vi "nonlinearmixpart.vi"(0 "Number of Samples":dbl, 1 "LO Frequency":dbl, 4 "Integer Degree of Nonlinearity (LO) (N) ( y(t) = x^1(t) + ...  + x^N(t) )":i32, 5 "Low Side / High Side":bool, 6 "Sampling Info":cluster{"Numeric 2":dbl, "Numeric":dbl}, 7 "RF Passband Bandwidth (Hz)":dbl, 9 "LO Gain Terms  (first gain term applied to linear part)":dbl[](array[numeric]), 10 "RF Carrier Frequency":dbl, 11 "Show Image Band":bool, 12 "Integer Degree of Nonlinearity (RF) (N) ( y(t) = x^1(t) + ...  + x^N(t) )":i32, 13 "RF Gain Terms (first gain term applied to linear part)":dbl[](array[numeric]), 19 "Duration (Seconds)":dbl) -> (14 "Post Distortion Passband Waveform":waveform(dbl), 15 "Post-distortion Local Oscillator Waveform":waveform(dbl), 17 "Pre-distortion passband waveform":waveform(dbl), 18 "Pre-distortion Local Oscillator Waveform":waveform(dbl))   [LabVIEW 2009]
uses:
  <vilib>/measure/NI_MABase.lvlib
  <vilib>/Analysis/NI_AALBase.lvlib
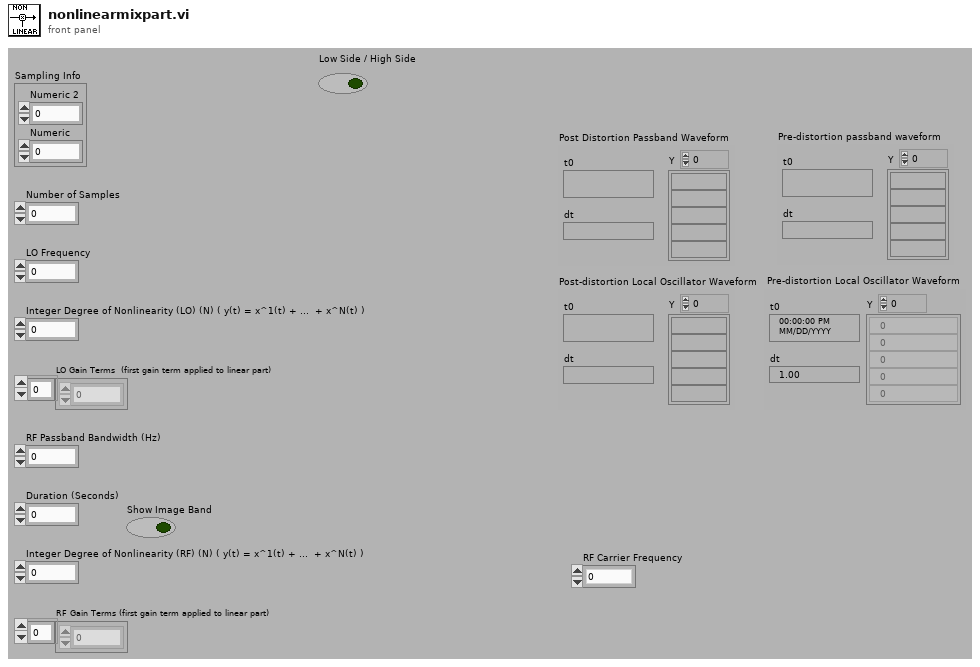
[diagram p1: front panel]
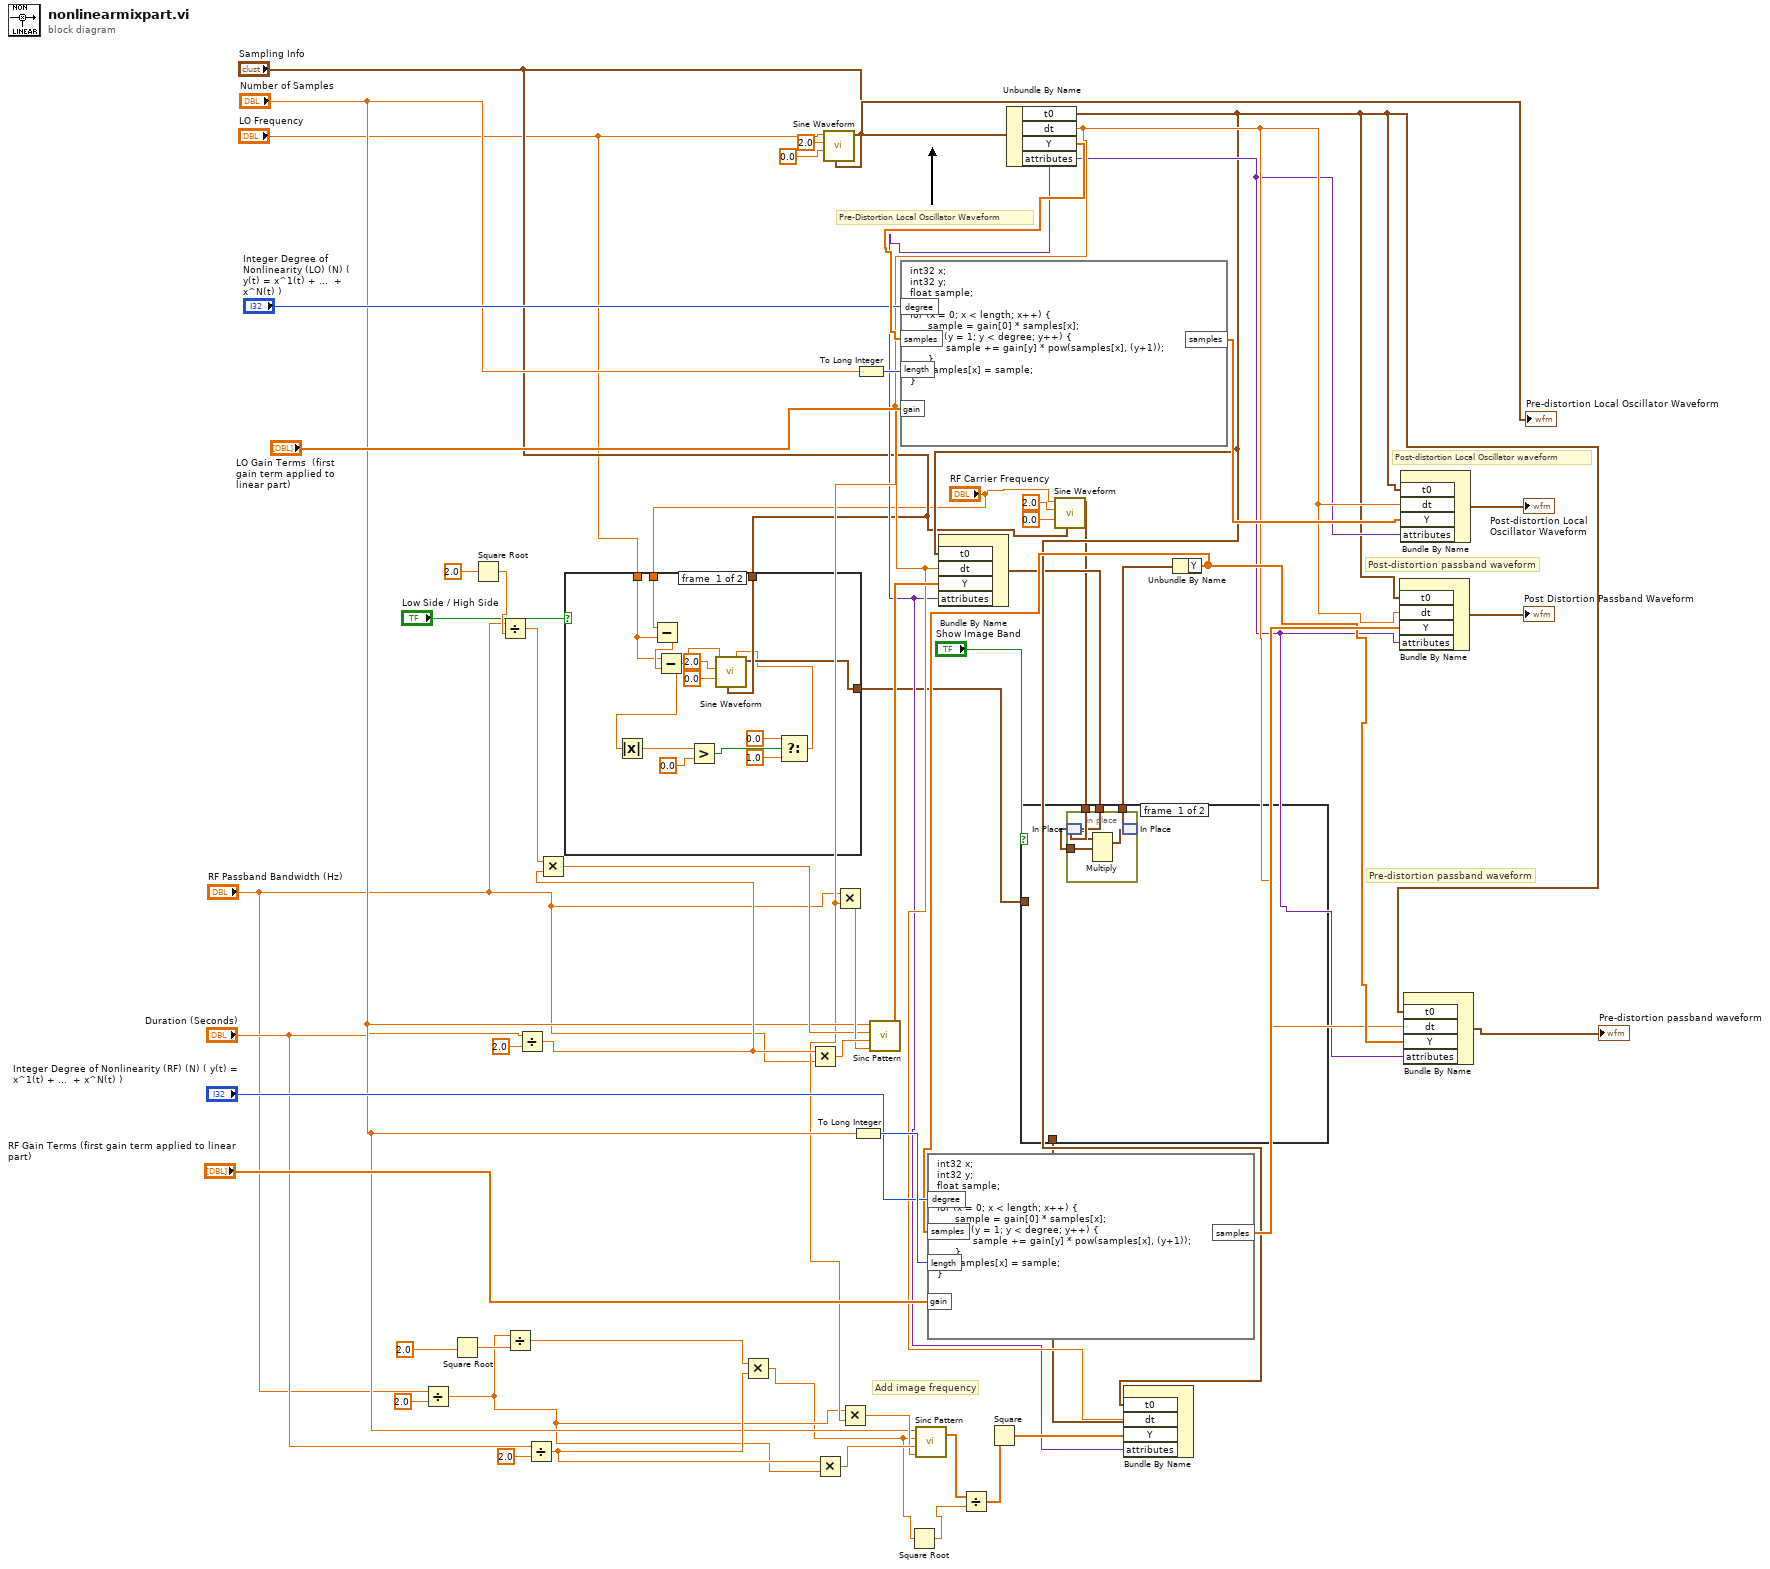
[diagram p0: block diagram]
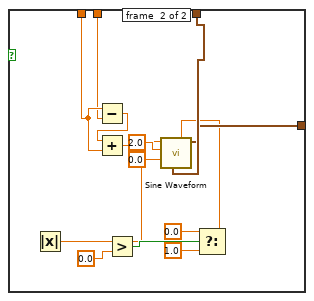
[diagram p2: hidden frame]
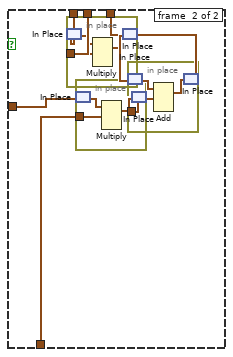
[diagram p3: hidden frame]
diagram:
  # "Add image frequency"
  # "Pre-Distortion Local Oscillator Waveform"
  # "Post-distortion Local Oscillator waveform"
  # "Post-distortion passband waveform"
  # "Pre-distortion passband waveform"
  n1 = Divide(x="RF Passband Bandwidth (Hz)", y=2.0) -> (x/y=w8:dbl)
  n2 = Square Root(x=2.0) -> (sqrt(x)=w28:dbl)
  n3 = Square Root(x=2.0) -> (sqrt(x)=w32:dbl)
  n4 = Divide(x="RF Passband Bandwidth (Hz)", y=w32) -> (x/y=w36:dbl)
  n5 = Divide(x=w8, y=w28) -> (x/y=w27:dbl)
  n6 = Divide(x="Duration (Seconds)", y=2.0) -> (x/y=w35:dbl)
  n7 = Divide(x="Duration (Seconds)", y=2.0) -> (x/y=w26:dbl)
  n8 = Multiply(x=w36, y=w35) -> (x*y=w34:dbl)
  n9 = case shown="True" "Low Side / High Side" {
    tunnel: "Sampling Info" -> [w69 w83]
    tunnel: "LO Frequency" -> [w66 w80]
    tunnel: "RF Carrier Frequency" -> [w68 w79]
    tunnel: [w63 w82] -> w10
    frame #0 {
      n10 = Subtract(x=w68, y=w66) -> (x-y=w67:dbl)
      n11 = Subtract(x=w66, y=w67) -> (x-y=w59:dbl)
      n12 = Absolute Value(x=w59) -> (abs(x)=w58:dbl)
      n13 = Greater?(x=w58, y=0.0) -> (0:w64:bool)
      n14 = Select(t=0.0, s=w64, f=1.0) -> (s? t:f=w62:dbl)
      n15 = call <vilib>:"Sine Waveform.vi"("offset"=w62, "sampling info"=w69, "phase"=0.0, "amplitude"=2.0, "frequency"=w59) -> ("signal out"=w63:waveform(dbl))  [unwired: 5 in, 1 out]
    }
    frame #1 {
      n16 = Subtract(x=w80, y=w79) -> (x-y=w81:dbl)
      n17 = Add(x=w81, y=w80) -> (x+y=w73:dbl)
      n18 = Absolute Value(x=w73) -> (abs(x)=w74:dbl)
      n19 = Greater?(x=w74, y=0.0) -> (0:w77:bool)
      n20 = Select(t=0.0, s=w77, f=1.0) -> (s? t:f=w72:dbl)
      n21 = call <vilib>:"Sine Waveform.vi"("offset"=w72, "sampling info"=w83, "phase"=0.0, "amplitude"=2.0, "frequency"=w73) -> ("signal out"=w82:waveform(dbl))  [unwired: 5 in, 1 out]
    }
  }
  n22 = Multiply(x=w27, y=w26) -> (x*y=w4:dbl)
  n23 = Multiply(x=w35, y="RF Passband Bandwidth (Hz)") -> (x*y=w56:dbl)
  n24 = Multiply(x=w26, y=w8) -> (x*y=w31:dbl)
  n25 = call <vilib>:"Sine Waveform.vi"("sampling info"="Sampling Info", "phase"=0.0, "amplitude"=2.0, "frequency"="LO Frequency") -> ("signal out"=w47:waveform(dbl))  [unwired: 6 in, 1 out]
  "Pre-distortion Local Oscillator Waveform" <- w47
  n26 = To Long Integer(number="Number of Samples") -> (32bit integer=w53:i32)
  n27 = To Long Integer(number="Number of Samples") -> (32bit integer=w44:i32)
  n28 = Square Root(x=w4) -> (sqrt(x)=w3:dbl)
  n29 = Unbundle By Name(w47) -> ("t0"=w19:timestamp, "dt"=w21:dbl, "Y"=w50:dbl[], "attributes"=w20:variant)
  n30 = Multiply(x="RF Passband Bandwidth (Hz)", y=w21) -> (x*y=w37:dbl)
  n31 = Multiply(x=w8, y=w21) -> (x*y=w29:dbl)
  n32 = call <vilib>:"Sinc Pattern.vi"("delta t"=w37, "delay"=w56, "amplitude"=w34, "samples"="Number of Samples") -> ("Sinc Pattern"=w41:dbl[])  [unwired: 1 out]
  n33 = formula code="int32 x;\nint32 y;\nfloat sample;\n\nfor (x = 0; x < length; x++) {\n      sample = gain[0] * samples[x];\n      for (y = 1; y < degree; y++) {\n            sample += gain[y] * pow(samples[x], (y+1));  \n      }\n      samples[x] = sample;\n}"("degree"="Integer Degree of Nonlinearity (LO) (N) ( y(t) = x^1(t) + ...  + x^N(t) )", "samples"=w50, "length"=w44, "gain"="LO Gain Terms  (first gain term applied to linear part)") -> ("samples"=w51:dbl[])
  n34 = call <vilib>:"Sinc Pattern.vi"("delta t"=w29, "delay"=w31, "amplitude"=w4, "samples"="Number of Samples") -> ("Sinc Pattern"=w6:dbl[])  [unwired: 1 out]
  n35 = Bundle By Name("t0"=w19, "dt"=w21, "Y"=w41, "attributes"=w20) -> (w15:waveform(dbl))  [unwired: 1 in]
  n36 = Divide(x=w6, y=w3) -> (x/y=w5:dbl[])
  n37 = Square(x=w5) -> (x^2=w22:dbl[])
  n38 = call <vilib>:"Sine Waveform.vi"("sampling info"="Sampling Info", "phase"=0.0, "amplitude"=2.0, "frequency"="RF Carrier Frequency") -> ("signal out"=w14:waveform(dbl))  [unwired: 6 in, 1 out]
  n39 = Bundle By Name("t0"=w19, "dt"=w21, "Y"=w22, "attributes"=w20) -> (w17:waveform(dbl))  [unwired: 1 in]
  n40 = case shown="True" "Show Image Band" {
    tunnel: w17 -> [_ w96]
    tunnel: w15 -> [w86 w97]
    tunnel: [w88 w93] -> w16
    tunnel: w14 -> [w87 w98]
    tunnel: w10 -> [_ w92]
    frame #0 {
      n41 = in-place {
        in-place-border: w86 -> [w89]
        n42 = in-place-match #1(w87) -> (w90:waveform(dbl))
        n43 = Multiply(1:w89, 2:w90) -> (0:w91:waveform(dbl))  [unwired: 1 in, 1 out]
        n44 = in-place-match #1(w91) -> (w88:waveform(dbl))
      }
    }
    frame #1 {
      n45 = in-place {
        in-place-border: w97 -> [w100]
        n46 = in-place-match #2(w98) -> (w101:waveform(dbl))
        n47 = Multiply(1:w100, 2:w101) -> (0:w99:waveform(dbl))  [unwired: 1 in, 1 out]
        n48 = in-place-match #2(w99) -> (w94:waveform(dbl))
      }
      n49 = in-place {
        in-place-border: w96 -> [w104]
        n50 = in-place-match #3(w92) -> (w102:waveform(dbl))
        n51 = Multiply(1:w104, 2:w102) -> (0:w103:waveform(dbl))  [unwired: 1 in, 1 out]
        n52 = in-place-match #3(w103) -> (w95:waveform(dbl))
      }
      n53 = in-place {
        in-place-border: w95 -> [w107]
        n54 = in-place-match #4(w94) -> (w106:waveform(dbl))
        n55 = Add(1:w107, 2:w106) -> (0:w105:waveform(dbl))  [unwired: 1 in, 1 out]
        n56 = in-place-match #4(w105) -> (w93:waveform(dbl))
      }
    }
  }
  n57 = Unbundle By Name(w16) -> ("Y"=w38:dbl[])
  n58 = formula code="int32 x;\nint32 y;\nfloat sample;\n\nfor (x = 0; x < length; x++) {\n      sample = gain[0] * samples[x];\n      for (y = 1; y < degree; y++) {\n            sample += gain[y] * pow(samples[x], (y+1));  \n      }\n      samples[x] = sample;\n}"("degree"="Integer Degree of Nonlinearity (RF) (N) ( y(t) = x^1(t) + ...  + x^N(t) )", "samples"=w38, "length"=w53, "gain"="RF Gain Terms (first gain term applied to linear part)") -> ("samples"=w57:dbl[])
  n59 = Bundle By Name("t0"=w19, "dt"=w21, "Y"=w57, "attributes"=w20) -> (→"Post Distortion Passband Waveform":waveform(dbl))  [unwired: 1 in]
  n60 = Bundle By Name("t0"=w19, "dt"=w21, "Y"=w51, "attributes"=w20) -> (→"Post-distortion Local Oscillator Waveform":waveform(dbl))  [unwired: 1 in]
  n61 = Bundle By Name("t0"=w19, "dt"=w21, "Y"=w38, "attributes"=w20) -> (→"Pre-distortion passband waveform":waveform(dbl))  [unwired: 1 in]
